vi "Point_Write.vi"   [LabVIEW 2017, in "PointValueMap.lvlib"]
doc: "Sets the value of a map point. If the point does not exist, you can optionally create the point. Wire data to the <B>Value</B> input to determine the polymorphic instance to use."
uses:
  <vilib>/addons/PointValueMap/PointValueMap.lvlib
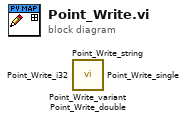
[diagram p0: block diagram]
diagram:
  n1 = call <vilib>:"Point_Write_variant.vi"() -> ()  [unwired: 10 in, 2 out]
  n2 = call <vilib>:"Point_Write_string.vi"() -> ()  [unwired: 10 in, 2 out]
  n3 = call <vilib>:"Point_Write_i32.vi"() -> ()  [unwired: 10 in, 2 out]
  n4 = call <vilib>:"Point_Write_single.vi"() -> ()  [unwired: 10 in, 2 out]
  n5 = call <vilib>:"Point_Write_double.vi"() -> ()  [unwired: 10 in, 2 out]
